vi "FTW-TestExecutive-Core_OnSequenceComplete.vi"(0 "FTW-TestExecutive-Core In":refnum<class "FTW-TestExecutive-Core.lvclass">, 11 "error in":errorcluster) -> (4 "FTW-TestExecutive-Core Out":refnum<class "FTW-TestExecutive-Core.lvclass">, 15 "error out":errorcluster)   [LabVIEW 2018, in "FTW-TestExecutive-Core.lvclass"]
uses:
  FTW-TestExecutive-Core.lvclass
  C:/Jobs/Featherweight/featherweight-2018/source/actor/Instance/FTW-ActorInstance.lvclass
  JSON/FTW-JSON-JoinMode.ctl
  FTW-TestExecutive-Core.lvclass/FTW-TestExecutive-Core.ctl
  c478ff23-f990-42a6-bfde-ed5cd6cf17a0.vi
  c478ff23-f990-42a6-bfde-ed5cd6cf17a0.vi/2ae51141-2f8f-4f15-93bb-5ed2a5a17510.vi
  container/FTW-Container-FromVariant.vi
  container/FTW-Container-New-FromContainer.vi
  JSON/FTW-JSON-SerializeAndDestroy.vi
  Instance/FTW-ActorInstance.lvclass
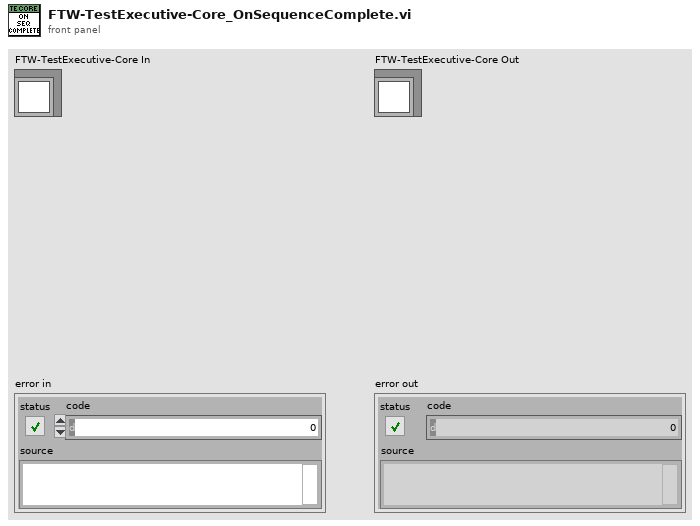
[diagram p1: front panel]
types:
  T1 = typedef "FTW-JSON-JoinMode.ctl" = enum32{"Upsert", "Update Only", "Insert Only"}
  T2 = typedef "FTW-TestExecutive-Step.ctl" = cluster{"Name":string, "Type":string, "Config":string, "Elapsed Time":dbl, "Passed":bool, "State":T3, "Results":T4}
  T3 = typedef "FTW-TestExecutive-Step-State.ctl" = enum8{"None", "Failed", "Passed", "Timed out", "Aborted"}
  T4 = typedef "FTW-TestExecutive-Results.ctl" = cluster{"Start Time":timestamp, "Elapsed Time":dbl, "Passed":bool, "Additional Results":string}
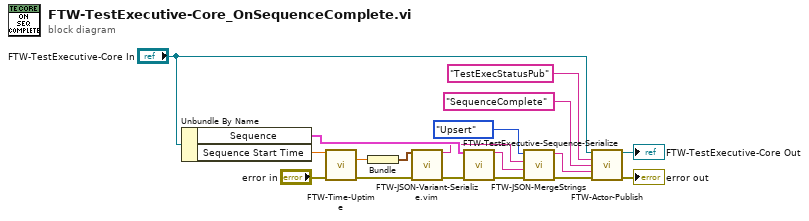
[diagram p0: block diagram]
diagram:
  n1 = Unbundle By Name("FTW-TestExecutive-Core In") -> ("Sequence"=w6:T2[], "Sequence Start Time"=w11:dbl)
  n2 = call "FTW-Time-Uptime.vi"("Previous Uptime"=w11, "error in"="error in") -> ("Elapsed Time"=w5:dbl, "error out"=w13:errorcluster)  [unwired: 11 in, 1 out]
  n3 = Bundle("Elapsed Time"=w5) -> (w1:cluster{"Elapsed Time":dbl})  [unwired: 1 in]
  n4 = call "FTW-JSON-Variant-Serialize.vim"("Variant"=w1, "error in"=w13) -> ("JSON String"=w3:string, "error out"=w8:errorcluster)  [unwired: 12 in]
  n5 = call "FTW-TestExecutive-Sequence-Serialize.vi"("Sequence"=w6, "error in"=w8) -> ("JSON"=w4:string, "error out"=w9:errorcluster)  [unwired: 12 in]
  n6 = call "FTW-JSON-MergeStrings.vi"("error in (no error)"=w9, "Initial JSON String (\"\")"=w4, "JSON string to merge (\"\")"=w3, "Update Mode (0: Upsert)"=FTW-JSON-JoinMode."Upsert") -> ("error out"=w10:errorcluster, "Merged JSON String (UTF-8)"=w2:string)  [unwired: 6 in]
  n7 = call "FTW-Actor-Publish.vi"("FTW-ActorExtended In"="FTW-TestExecutive-Core In", "Publisher Name"="TestExecStatusPub", "Message Header"="SequenceComplete", "Message Body"=w2, "error in"=w10) -> ("FTW-ActorExtended Out"=→"FTW-TestExecutive-Core Out":refnum<class "FTW-TestExecutive-Core.lvclass">, "error out"=→"error out":errorcluster)  [unwired: 9 in]
